vi "Get Attributes.vi"(8 "error in (no error)":errorcluster, 11 "Noise in":refnum<class "Noise.lvclass">) -> (0 "error out":errorcluster, 2 "Attributes":T1={"Spectrum"=TRUE, "Gate"=TRUE, "Mod"=TRUE, "Filter"=TRUE}, 3 "Noise out":refnum<class "Noise.lvclass">)   [LabVIEW 2020, in "Noise.lvclass"]
uses:
  Noise.lvclass
  Waveform/Attributes.ctl
  Waveform/Waveform.lvclass
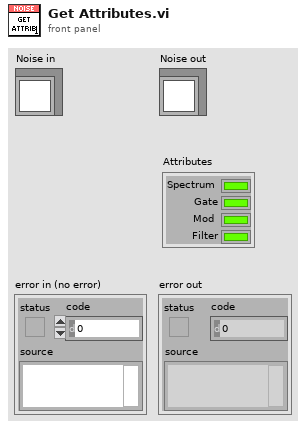
[diagram p1: front panel]
types:
  T1 = typedef "Waveform.lvclass/Attributes.ctl" = cluster{"Spectrum":bool, "Gate":bool, "Mod":bool, "Filter":bool}
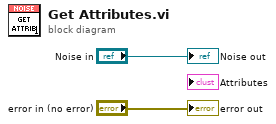
[diagram p0: block diagram]
diagram:
  "error out" <- "error in (no error)"
  "Noise out" <- "Noise in"
